vi "CANOpen Addon RT Driver VI.vi"(7 "Operation":T1, 11 "Device Reference in":T2 format="%.0x") -> (0 "Error Code":i32)   [LabVIEW 2013, in "CANOpen Addon Custom Device.lvlib"]
uses:
  CANOpen Addon Custom Device.lvlib
  <vilib>/NI Veristand/Custom Device API/Custom Device Item Ref.ctl
  <vilib>/NI Veristand/Custom Device API/Hardware Interface Driver VI Operation.ctl
  SubVIS/Inline Async API/_Controls/Async VI Control_Parameters Cluster.ctl
  SubVIS/Error Handling API/_Controls/VS Errors_Error Handling Cluster.ctl
  SubVIS/CANOpen_Settings.ctl
  SubVIS/CANOpen_Node Settings.ctl
  Shared Code/CANOpen_Bus Settings.ctl
  Shared Code/CANOpen Interface Name.ctl
  <vilib>/CANopenLib/CANOPEN.llb/CANopen BaudRate.ctl
  SubVIS/CANOpen_Node Message Settings.ctl
  Shared Code/CANOpen_PDO Settings.ctl
  Shared Code/CANOpen_PDO Parameter Settings.ctl
  Shared Code/CANOpen_PDO Data Type.ctl
  System Explorer/SubVIs/CANopen Byte Order.ctl
  Shared Code/CANOpen_SDO Settings.ctl
  SubVIS/CANOpen_NMT Settings.ctl
  Async VIs/CANOpen_Main/SubVIs/CanOpen_NMT_Config.ctl
  Async VIs/CANOpen_Main/SubVIs/CanOpen_NMT_Static detect.ctl
  Async VIs/CANOpen_Main/SubVIs/CanOpen_Main Node Ids.ctl
  SubVIS/CANOpen_VS Data Refs.ctl
  <vilib>/NI Veristand/Custom Device API/Data Reference.ctl
  <vilib>/NI Veristand/Custom Device API/Block Data Reference.ctl
  SubVIS/CANOpen_VS Bidirectional Data Refs.ctl
  SubVIS/CANOpen_VS SDOs Data Refs.ctl
  Async VIs/CANOpen_Main/SubVIs/CanOpen_SDO Dynamic queue.ctl
  Shared Code/CANOpen_SDO queue W data.ctl
  Shared Code/CANOpen_SDO queue mode.ctl
  Shared Code/CANOpen_PDO Data Type in queue.ctl
  SubVIS/CANOpen_VS Status Management Data Refs.ctl
  Async VIs/CANOpen_Main/SubVIs/CanOpen_NMT_HWOut_ChannelPairs.ctl
  Async VIs/CANOpen_Main/SubVIs/CanOpen_NMT_HWIn_ChannelPairs.ctl
  SubVIS/CANOpen_Get xPDO Data Refs.vi
  Shared Code/CANOpen_Get Node ID from Name.vi
  SubVIS/CANOpen_Get SDOs Settings.vi
  SubVIS/CANOpen_Get Dynamic SDOs Settings.vi
  SubVIS/CANOpen_NMR Read config.vi
  SubVIS/CANOpen_SetGet Bus Settings.vi
  SubVIS/CANOpen_Get Section References by GUID.vi
  SubVIS/CANOpen_Initialize VS Data Refs.vi
  SubVIS/CANOpen_Get Section References by GUID for SDOs.vi
  SubVIS/CANOpen_Get Section References by GUID for NMT.vi
  <vilib>/NI Veristand/Custom Device API/NI VeriStand - Set Channel Value by Data Reference.vi
  <vilib>/NI Veristand/Custom Device API/NI VeriStand - Get Channel Value by Data Reference.vi
  SubVIS/CANOpen_SDO List RW.vi
  SubVIS/CANOpen_SDO Read RW.vi
  SubVIS/CANOpen_SDO Write RW.vi
  <vilib>/NI Veristand/Custom Device API/NI VeriStand - Get Channel Values by Block Data Reference.vi
  <vilib>/NI Veristand/Custom Device API/NI VeriStand - Set Channel Values by Block Data Reference.vi
  SubVIS/Error Handling API/Print/VS Errors_Display and Log Custom Device Error.vi
  Shared Code/CANOpen_Get PDO Channel from Name.vi
  Shared Code/CANOpen_SetGet PDO Parameter Settings.vi
  SubVIS/CANOpen_SetGet NMT Settings.vi
  SubVIS/CANOpen_Initialize VS BiDirectional Data Refs.vi
  SubVIS/CANOpen_Search Channel Ref.vi
  SubVIS/CANOpen_Search Channel Refs.vi
  SubVIS/CANOpen_Initialize VS NMT Data Refs.vi
  SubVIS/CANOpen_SDO Update status channels Dyn Read.vi
  SubVIS/CANOpen_SDO Update status channels Dyn Write.vi
  <vilib>/NI Veristand/Custom Device Tools/Custom Device Utility Library/NI VeriStand - Search for Item.vi
  <vilib>/NI Veristand/Custom Device Tools/Custom Device Utility Library/NI VeriStand - Search for All Items by GUID.vi
  <vilib>/NI Veristand/Custom Device API/NI VeriStand - Get Item Property.vi
  <vilib>/NI Veristand/Custom Device API/Get Item Property (Variant).vi
  Shared Code/CANOpen Addon GUID Lookup Global.vi
  <vilib>/NI Veristand/Custom Device API/NI VeriStand - Get Item Children.vi
  <vilib>/NI Veristand/Custom Device Tools/Custom Device Utility Library/NI VeriStand - Search for Item by GUID.vi
  <vilib>/NI Veristand/Custom Device API/NI VeriStand - Get Channel Data Reference.vi
  <vilib>/NI Veristand/Custom Device API/NI VeriStand - Get Channel Block Data References.vi
  <vilib>/NI Veristand/Custom Device API/Global Data Refs.vi
  <vilib>/Utility/error.llb/Simple Error Handler.vi
  <vilib>/NI Veristand/Custom Device API/Custom Device API.lvlib
  <vilib>/NI Veristand/Custom Device API/Custom Device Item Info.ctl
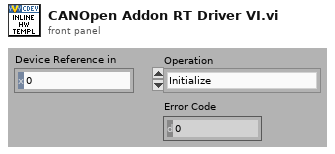
[diagram p1: front panel]
types:
  T1 = typedef "Custom Device API.lvlib/Hardware Interface Driver VI Operation.ctl" = enum16{"Initialize", "Start", "Read Data from HW", "Write Data to HW", "Close"}
  T2 = typedef "Custom Device API.lvlib/Custom Device Item Ref.ctl" = u64
  T3 = typedef "CANOpen Addon Custom Device.lvlib/VS Errors_Error Handling Cluster.ctl" = cluster{"Error Process Q":refnum<queue>, "Process Qs":refnum<queue>[]}
  T4 = typedef "CANOpen_Settings.ctl" = cluster{"Driver Settings":T5, "Data References":T19, "Bus Commands":T22, "SDO Asynch":T23, "Status NMT":T24}
  T5 = typedef "CANOpen_Node Settings.ctl" = cluster{"CANOpen Bus Settings":T6, "Nodes":T9[], "Node Ids":T18}
  T6 = typedef "CANOpen Addon Custom Device.lvlib/CANOpen_Bus Settings.ctl" = cluster{"CANOpen Interface Name":T7, "Baud Rate":T8, "Termination":bool, "Sync Period (ms)":i64, "Enable 9881":bool, "RIO Device":u16, "Enable SYNC":bool, "Scan & Print":bool}
  T7 = typedef "CANOpen Addon Custom Device.lvlib/CANOpen Interface Name.ctl" = u32
  T8 = typedef "CANopen BaudRate.ctl" = u32
  T9 = typedef "CANOpen_Node Message Settings.ctl" = cluster{"RPDOs":T10[], "TPDOs":T10[], "Node ID":u8, "SDOs":T14[], "Dynamic SDOs":T14[], "NMT":T15}
  T10 = typedef "CANOpen Addon Custom Device.lvlib/CANOpen_PDO Settings.ctl" = cluster{"Parameters":T11[], "PDO Channel":u8, "Start Index":u32, "Length":u32}
  T11 = typedef "CANOpen Addon Custom Device.lvlib/CANOpen_PDO Parameter Settings.ctl" = cluster{"Parameter Name":string, "Scale Factor":dbl, "Scale Offset":dbl, "Byte Offset":u8, "Bit Offset":u8, "Data Type":T12, "Byte Order":T13}
  T12 = typedef "CANOpen Addon Custom Device.lvlib/CANOpen_PDO Data Type.ctl" = enum16{"U8", "U16", "U32", "I8", "I16", "I32", "Single", "Double", "Boolean"}
  T13 = typedef "CANOpen Addon Custom Device.lvlib/CANopen Byte Order.ctl" = enum16{"big-endian network order", "little-endian"}
  T14 = typedef "CANOpen Addon Custom Device.lvlib/CANOpen_SDO Settings.ctl" = cluster{"Object Index":u16, "Sub-Index (0)":u8, "Block Data":u8[], "Name":string}
  T15 = typedef "CANOpen Addon Custom Device.lvlib/CANOpen_NMT Settings.ctl" = cluster{"Node run state":u16, "Emergency":bool, "HB NG":T16, "Delay for opp. state (ms)":dbl, "Node init static SDO state":u16, "Stop and Reset on Shutdown":bool}
  T16 = typedef "CANOpen Addon Custom Device.lvlib/CanOpen_NMT_Config.ctl" = cluster{"Mode":T17, "Update Time":u16, "Static detect in None":T17}
  T17 = typedef "CANOpen Addon Custom Device.lvlib/CanOpen_NMT_Static detect.ctl" = enum16{"None", "HB", "NG"}
  T18 = typedef "CANOpen Addon Custom Device.lvlib/CanOpen_Main Node Ids.ctl" = u8[]
  T19 = typedef "CANOpen_VS Data Refs.ctl" = cluster{"Hardware Input":cluster{"FIFO":refnum<k33>, "Channel Pairs":cluster{"Chan Refs":T20[], "Prev. Values":dbl[]}}, "Hardware Output":cluster{"FIFO":refnum<k33>, "Channel Pairs":cluster{"Block Refs":T21[], "Prev. Values":dbl[]}}}
  T20 = typedef "Custom Device API.lvlib/Data Reference.ctl" = i32
  T21 = typedef "Custom Device API.lvlib/Block Data Reference.ctl" = cluster{"Data Reference":T20, "Offset":i32, "Length":i32}
  T22 = typedef "CANOpen_VS Bidirectional Data Refs.ctl" = cluster{"Hardware Output":cluster{"FIFO":refnum<k33>, "Channel Pairs":cluster{"Chan Refs":T20[], "Prev. Values":dbl[]}}, "Hardware Input":cluster{"FIFO":refnum<k33>}}
  T23 = typedef "CANOpen Addon Custom Device.lvlib/CANOpen_VS SDOs Data Refs.ctl" = cluster{"List SDO":cluster{"FIFO Req":refnum<k33>, "Req Chan.":cluster{"Chan Refs":T20[], "NodeIndex":dbl[]}, "FIFO Resp":refnum<k33>, "Resp Chan.":cluster{"Chan Refs":T20[]}, "Node IDs":u8[], "FIFO array":dbl[]}, "HW Dyn Write":cluster{"FIFO Req":refnum<k33>, "FIFO Resp":refnum<k33>, "Req Chan.":cluster{"Chan Refs":T20[], "Node IDs":u8[]}, "Resp Chan.":cluster{"Chan Refs":T20[]}}, "HW Dyn Read":cluster{"FIFO Req":refnum<k33>, "FIFO Resp":refnum<k33>, "Req Chan.":cluster{"Chan Refs":T20[], "Node IDs":u8[]}, "Resp Chan.":cluster{"Chan Refs":T20[]}}}
  T24 = typedef "CANOpen Addon Custom Device.lvlib/CANOpen_VS Status Management Data Refs.ctl" = cluster{"Hardware Output":cluster{"FIFO":refnum<k33>, "Channel Pairs":T25}, "Hardware Input":cluster{"FIFO":refnum<k33>, "Channel Pairs":T26}}
  T25 = typedef "CANOpen Addon Custom Device.lvlib/CanOpen_NMT_HWOut_ChannelPairs.ctl" = cluster{"Chan Refs":T21[], "Prev. Values":dbl[], "Node index":dbl[]}
  T26 = typedef "CANOpen Addon Custom Device.lvlib/CanOpen_NMT_HWIn_ChannelPairs.ctl" = cluster{"Chan Refs":T20[], "Prev. Values":dbl[], "Node index":dbl[]}
  T27 = cluster{"Device Error":errorcluster, "Error Handling Cluster":T3, "VI Ref In":refnum<vi>[], "CD Settings":T4, "FPGA Session":u32}
  T28 = typedef "CANOpen Addon Custom Device.lvlib/Async VI Control_Parameters Cluster.ctl" = cluster{"Parameter Name":string, "Initial Settings":variant}
  T29 = typedef "Custom Device API.lvlib/Custom Device Item Info.ctl" = cluster{"Name":string, "Is Channel":bool, "GUID":string, "Is Waveform":bool}
  T30 = cluster{"Chan Refs":T20[], "Previous Chan Values":dbl[]}
  T31 = cluster{"Block Refs":T21[], "Prev. Values":dbl[]}
  T32 = cluster{"Block Data Refs":T21[], "Previous Chan Values":dbl[]}
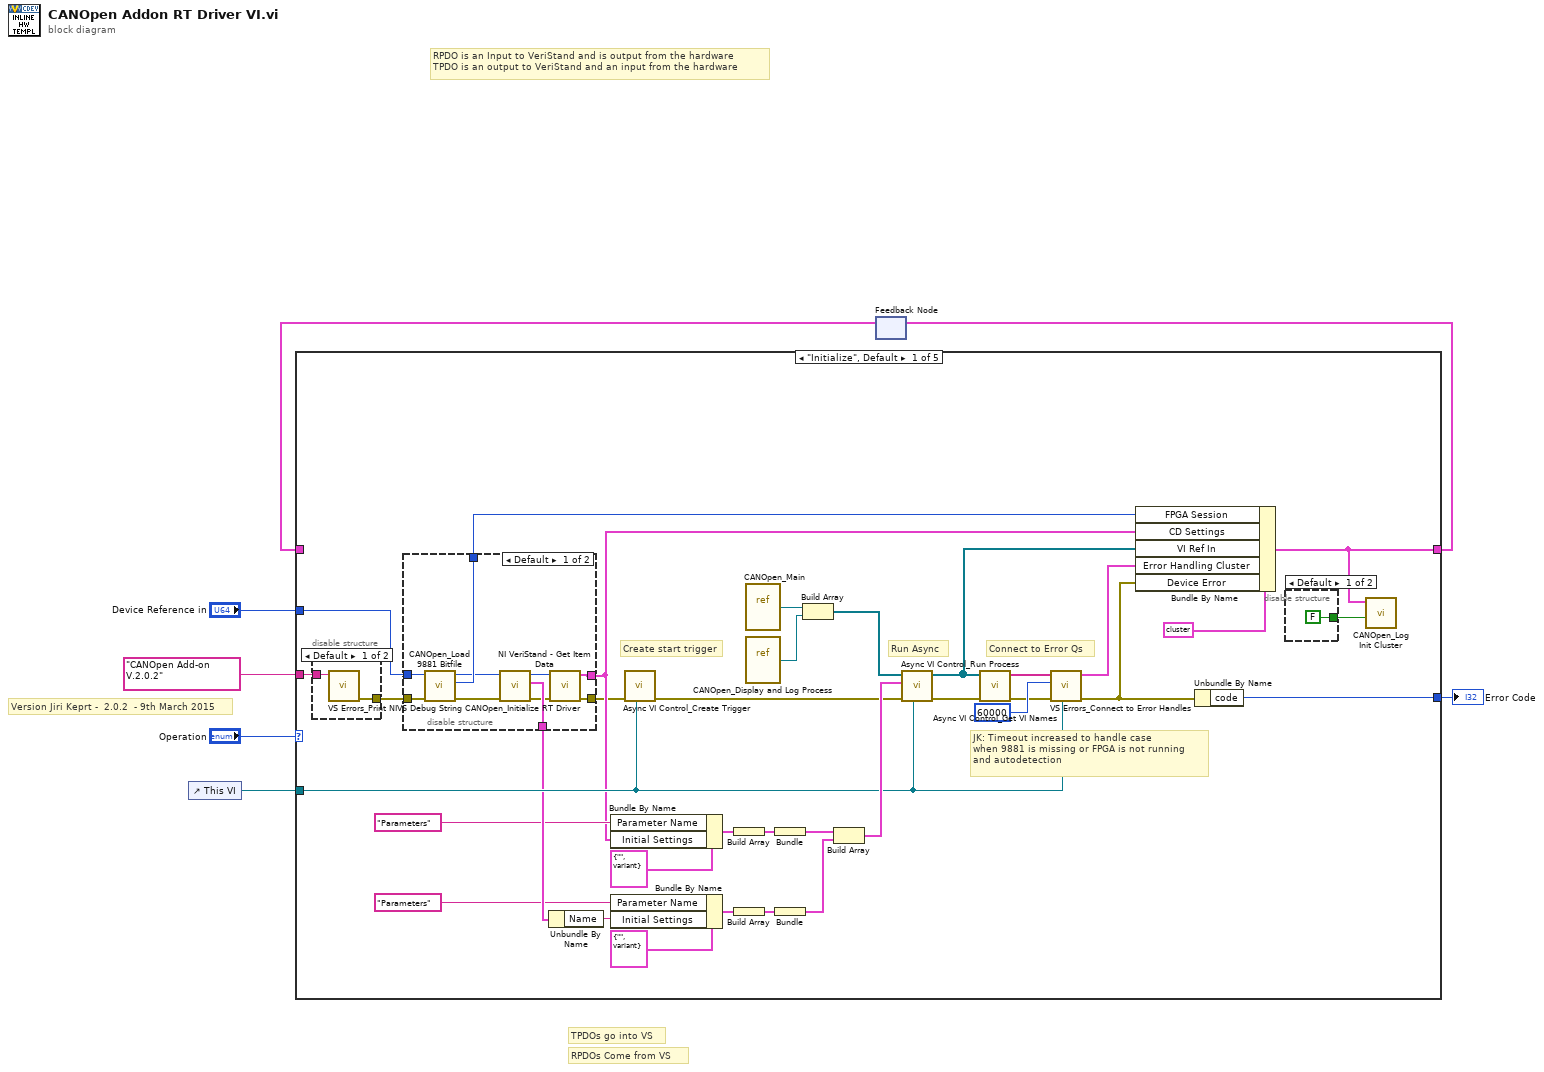
[diagram p0: block diagram]
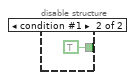
[diagram p2: hidden frame]
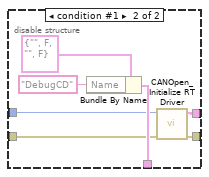
[diagram p4: hidden frame]
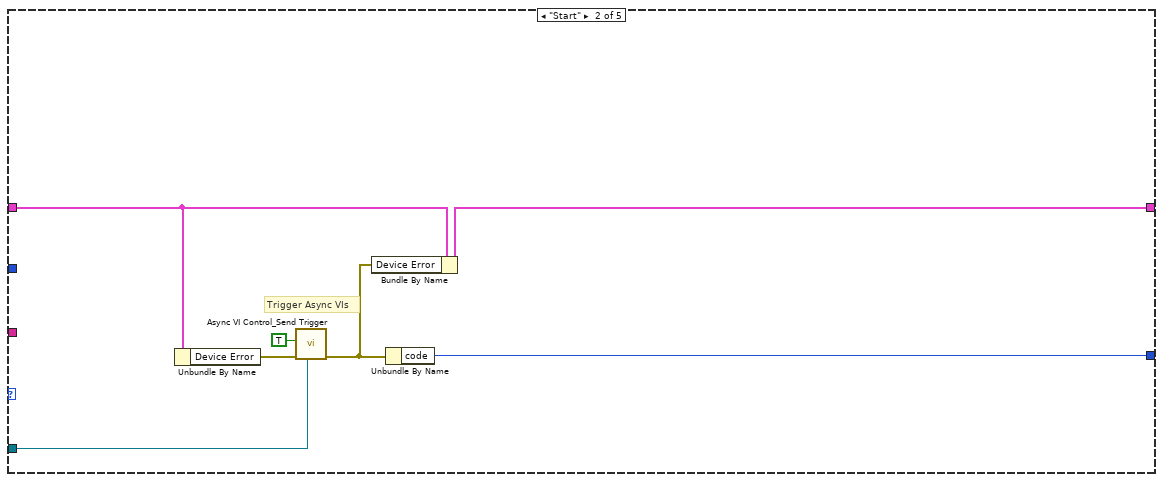
[diagram p5: hidden frame]
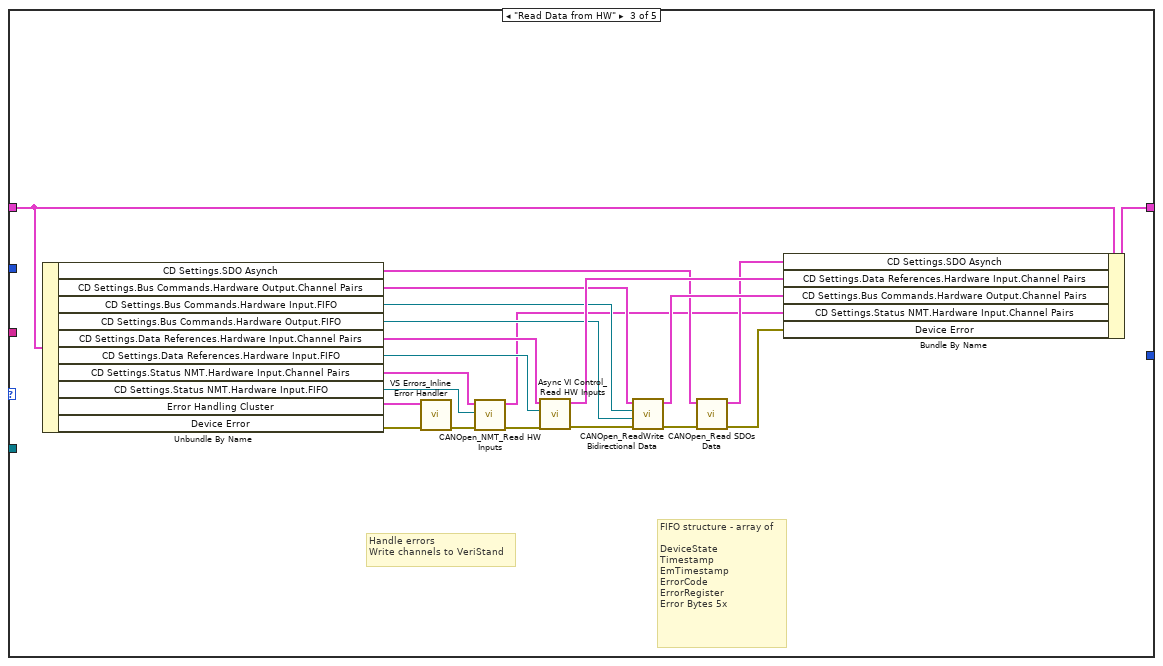
[diagram p6: hidden frame]
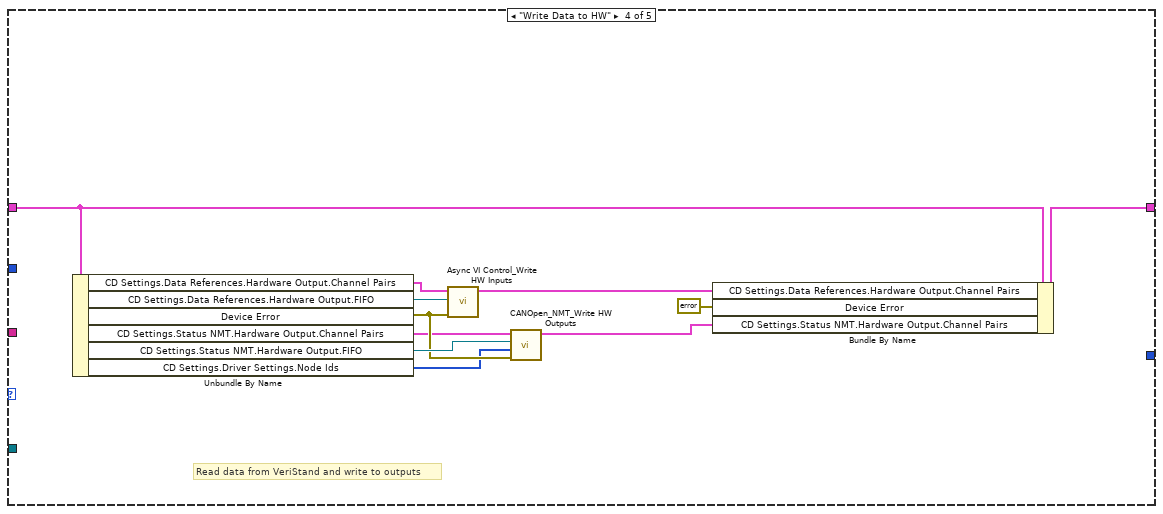
[diagram p7: hidden frame]
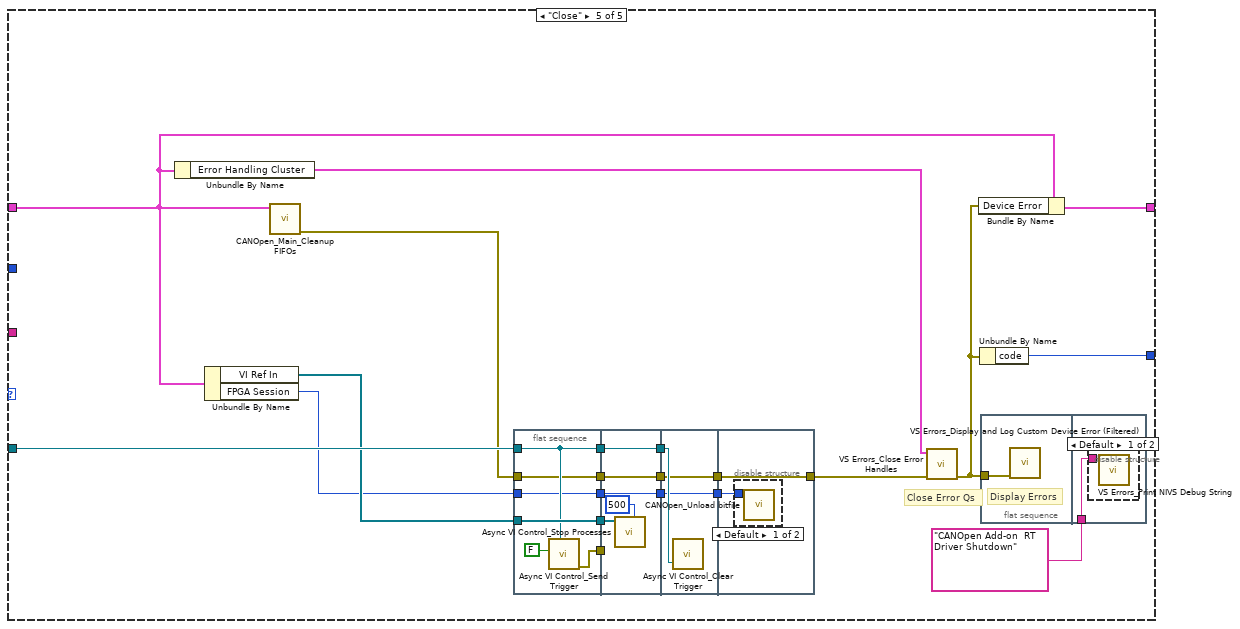
[diagram p8: hidden frame]
diagram:
  # "Version Jiri Keprt -  2.0.2  - 9th March 2015"
  # "RPDO is an Input to VeriStand and is output from the hardware\nTPDO is an output to VeriStand and an input from the hardware"
  # "RPDOs Come from VS"
  # "TPDOs go into VS"
  n1 = control-ref of="This VI"() -> (w1:refnum<vi>)
  n2 = feedback #1() -> (w5:T27)  [unwired: 1 out]
  n3 = case shown="\"Initialize\", Default" "Operation" {
    tunnel: [w19 w66 w87 w98 w122] -> w6
    tunnel: w5 -> [_ w67 w88 w99 w109]
    tunnel: "Device Reference in" -> [w15 _ _ _ _]
    tunnel: [w42 w65 _ _ w121] -> w3
    tunnel: "CANOpen Add-on  V.2.0.2" ("Debug String") -> [w41 _ _ _ _]
    tunnel: w1 -> [w30 w64 _ _ w113]
    frame "Initialize", Default {
      # "JK: Timeout increased to handle case\nwhen 9881 is missing or FPGA is not running\nand autodetection"
      # "Connect to Error Qs"
      # "Run Async"
      # "Create start trigger"
      n4 = disable-structure shown="Default" {
        disable-tunnel: w41 -> [w46 _]
        disable-tunnel: [w45 _] -> w13
        frame condition #0 (active) {
          n5 = call "VS Errors_Print NIVS Debug String.vi"("Debug String"=w46) -> ("error out"=w45:errorcluster)  [unwired: 9 in]
        }
        frame condition #1 {
        }
      }
      n6 = disable-structure shown="Default" {
        disable-tunnel: [w56 w61] -> w29
        disable-tunnel: [w54 w57] -> w17
        disable-tunnel: w15 -> [w53 w58]
        disable-tunnel: [w52 _] -> w14
        disable-tunnel: w13 -> [w50 w59]
        disable-tunnel: [w47 w60] -> w8
        frame condition #0 (active) {
          n7 = call "CANOpen_Load 9881 Bitfile.vi"("error in (no error)"=w50, "Item Ref in"=w53) -> ("error out"=w49:errorcluster, "FPGA Session"=w52:u32, "Item Ref out"=w51:T2)  [unwired: 7 in]
          n8 = call <vilib>:"NI VeriStand - Get Item Data.vi"("error in (no error)"=w49, "Item Ref in"=w51) -> ("error out"=w48:errorcluster, "Item Info"=w56:T29, "Item Ref out"=w55:T2)  [unwired: 6 in, 1 out]
          n9 = call "CANOpen_Initialize RT Driver.vi"("error in (no error)"=w48, "Device Reference in"=w55) -> ("error out"=w47:errorcluster, "Configuration Cluster"=w54:T4)  [unwired: 8 in]
        }
        frame condition #1 {
          n10 = Bundle By Name(cluster=T29 {"Name"="", "Is Channel"=FALSE, "GUID"="", "Is Waveform"=FALSE} ("Item Info"), "Name"="DebugCD") -> (w61:T29)
          n11 = call "CANOpen_Initialize RT Driver.vi"("error in (no error)"=w59, "Device Reference in"=w58) -> ("error out"=w60:errorcluster, "Configuration Cluster"=w57:T4)  [unwired: 8 in]
        }
      }
      n12 = Unbundle By Name(w29) -> ("Name"=w28:string)
      n13 = Bundle By Name(cluster=T28 {"Parameter Name"="", "Initial Settings"=variant} ("Parameters"), "Parameter Name"="Parameters", "Initial Settings"=w17) -> (w23:T28)
      n14 = Bundle By Name(cluster=T28 {"Parameter Name"="", "Initial Settings"=variant} ("Parameters"), "Parameter Name"="Parameters", "Initial Settings"=w28) -> (w37:T28)
      n15 = call "Async VI Control_Create Trigger.vi"("This VI"=w30, "error in (no error)"=w8) -> ("error out"=w12:errorcluster)  [unwired: 9 in]
      n16 = Build Array(w23) -> (w24:T28[])
      n17 = Build Array(w37) -> (w38:T28[])
      n18 = vi-ref "CANOpen_Main.vi"() -> (w35:refnum<vi>)
      n19 = vi-ref "CANOpen_Display and Log Process.vi"() -> (w31:refnum<vi>)
      n20 = Bundle ("Display and Log Process Parameters")(w24) -> (w20:cluster{T28[]})  [unwired: 1 in]
      n21 = Bundle ("Display and Log Process Parameters")(w38) -> (w39:cluster{T28[]})  [unwired: 1 in]
      n22 = Build Array(w35, w31) -> (w32:refnum<vi>[])
      n23 = Build Array(w20, w39) -> (w40:cluster{T28[]}[])
      n24 = call "Async VI Control_Run Process.vi"("Parent VI"=w30, "error in (no error)"=w12, "Initial Parameters"=w40, "VI Ref In"=w32) -> ("error out"=w11:errorcluster, "VI Ref In"=w25:refnum<vi>[])  [unwired: 6 in]
      n25 = call "Async VI Control_Get VI Names.vi"("error in"=w11, "VI References"=w25) -> ("error out"=w10:errorcluster, "Clone Names"=w33:string[])  [unwired: 8 in]
      n26 = call "VS Errors_Connect to Error Handles.vi"("Parent"=w30, "error in"=w10, "Timeout (ms)"=u16 60000, "Process Names"=w33) -> ("error out"=w9:errorcluster, "Error Handling Cluster"=w26:T3)  [unwired: 6 in]
      n27 = Bundle By Name(cluster=T27 {"Device Error"={"status"=FALSE, "code"=0, "source"=""}, "Error Handling Cluster"={"Error Process Q"=refnum, "Process Qs"=[]}, "VI Ref In"=[], "CD Settings"={"Driver Settings"={"CANOpen Bus Settings"={"CANOpen Interface Name"=0, "Baud Rate"=0, "Termination"=FALSE, "Sync Period (ms)"=0, "Enable 9881"=FALSE, "RIO Device"=0, "Enable SYNC"=FALSE, "Scan & Print"=FALSE}, "Nodes"=[], "Node Ids"=[]}, "Data References"={"Hardware Input"={"FIFO"=refnum, "Channel Pairs"={"Chan Refs"=[], "Prev. Values"=[]}}, "Hardware Output"={"FIFO"=refnum, "Channel Pairs"={"Block Refs"=[], "Prev. Values"=[]}}}, "Bus Commands"={"Hardware Output"={"FIFO"=refnum, "Channel Pairs"={"Chan Refs"=[], "Prev. Values"=[]}}, "Hardware Input"={"FIFO"=refnum}}, "SDO Asynch"={"List SDO"={"FIFO Req"=refnum, "Req Chan."={"Chan Refs"=[], "NodeIndex"=[]}, "FIFO Resp"=refnum, "Resp Chan."={"Chan Refs"=[]}, "Node IDs"=[], "FIFO array"=[]}, "HW Dyn Write"={"FIFO Req"=refnum, "FIFO Resp"=refnum, "Req Chan."={"Chan Refs"=[], "Node IDs"=[]}, "Resp Chan."={"Chan Refs"=[]}}, "HW Dyn Read"={"FIFO Req"=refnum, "FIFO Resp"=refnum, "Req Chan."={"Chan Refs"=[], "Node IDs"=[]}, "Resp Chan."={"Chan Refs"=[]}}}, "Status NMT"={"Hardware Output"={"FIFO"=refnum, "Channel Pairs"={"Chan Refs"=[], "Prev. Values"=[], "Node index"=[]}}, "Hardware Input"={"FIFO"=refnum, "Channel Pairs"={"Chan Refs"=[], "Prev. Values"=[], "Node index"=[]}}}}, "FPGA Session"=0}, "FPGA Session"=w14, "CD Settings"=w17, "VI Ref In"=w25, "Error Handling Cluster"=w26, "Device Error"=w9) -> (w19:T27)
      n28 = Unbundle By Name(w9) -> ("code"=w42:i32)
      n29 = disable-structure shown="Default" {
        disable-tunnel: [FALSE ("Write?") TRUE ("Write?")] -> w18
        frame condition #0 (active) {
        }
        frame condition #1 {
        }
      }
      n30 = call "CANOpen_Log Init Cluster.vi"("Write?"=w18, "cluster 2"=w19) -> ()  [unwired: 8 in, 2 out]
    }
    frame "Start" {
      # "Trigger Async VIs"
      n31 = Unbundle By Name(w67) -> ("Device Error"=w68:errorcluster)
      n32 = call "Async VI Control_Send Trigger.vi"("Parent VI"=w64, "error in (no error)"=w68, "notification"=TRUE) -> ("error out"=w69:errorcluster)  [unwired: 8 in]
      n33 = Bundle By Name(cluster=w67, "Device Error"=w69) -> (w66:T27)
      n34 = Unbundle By Name(w69) -> ("code"=w65:i32)
    }
    frame "Read Data from HW" {
      # "FIFO structure - array of\n\nDeviceState\nTimestamp\nEmTimestamp\nErrorCode\nErrorRegister\nError Bytes 5x"
      # "Handle errors\nWrite channels to VeriStand"
      n35 = Unbundle By Name(w88) -> ("CD Settings.SDO Asynch"=w80:T23, "CD Settings.Bus Commands.Hardware Output.Channel Pairs"=w84:cluster{"Chan Refs":T20[], "Prev. Values":dbl[]}, "CD Settings.Bus Commands.Hardware Input.FIFO"=w83:refnum<k33>, "CD Settings.Bus Commands.Hardware Output.FIFO"=w82:refnum<k33>, "CD Settings.Data References.Hardware Input.Channel Pairs"=w89:cluster{"Chan Refs":T20[], "Prev. Values":dbl[]}, "CD Settings.Data References.Hardware Input.FIFO"=w91:refnum<k33>, "CD Settings.Status NMT.Hardware Input.Channel Pairs"=w73:T26, "CD Settings.Status NMT.Hardware Input.FIFO"=w74:refnum<k33>, "Error Handling Cluster"=w77:T3, "Device Error"=w78:errorcluster)
      n36 = call "VS Errors_Inline Error Handler.vi"("error in"=w78, "Error Handling Cluster"=w77) -> ("error out"=w75:errorcluster)  [unwired: 9 in]
      n37 = call "CANOpen_NMT_Read HW Inputs.vi"("error in"=w75, "Hardware Input FIFO"=w74, "Channel Pairs"=w73) -> ("error out"=w76:errorcluster, "Channel Pairs Out"=w71:T26)  [unwired: 6 in, 1 out]
      n38 = call "Async VI Control_Read HW Inputs.vi"("error in"=w76, "Hardware Input FIFO"=w91, "Channel Pairs"=w89) -> ("error out"=w86:errorcluster, "Channel Pairs Out"=w90:T30)  [unwired: 6 in, 1 out]
      n39 = call "CANOpen_ReadWrite Bidirectional Data.vi"("error in"=w86, "Hardware Output FIFO"=w82, "Hardware Input FIFO"=w83, "Channel Pairs"=w84) -> ("error out"=w81:errorcluster, "Channel Pairs Out"=w85:T30)  [unwired: 5 in, 1 out]
      n40 = call "CANOpen_Read SDOs Data.vi"("error in"=w81, "SDO Asynch"=w80) -> ("error out"=w72:errorcluster, "SDO Asynch out"=w79:T23)  [unwired: 8 in]
      n41 = Bundle By Name(cluster=w88, "CD Settings.SDO Asynch"=w79, "CD Settings.Data References.Hardware Input.Channel Pairs"=w90, "CD Settings.Bus Commands.Hardware Output.Channel Pairs"=w85, "CD Settings.Status NMT.Hardware Input.Channel Pairs"=w71, "Device Error"=w72) -> (w87:T27)
    }
    frame "Write Data to HW" {
      # "Read data from VeriStand and write to outputs"
      n42 = Unbundle By Name(w99) -> ("CD Settings.Data References.Hardware Output.Channel Pairs"=w101:T31, "CD Settings.Data References.Hardware Output.FIFO"=w102:refnum<k33>, "Device Error"=w96:errorcluster, "CD Settings.Status NMT.Hardware Output.Channel Pairs"=w95:T25, "CD Settings.Status NMT.Hardware Output.FIFO"=w97:refnum<k33>, "CD Settings.Driver Settings.Node Ids"=w94:T18)
      n43 = call "Async VI Control_Write HW Inputs.vi"("error in"=w96, "Hardware Output FIFO"=w102, "Channel Pairs"=w101) -> ("Channel Pairs"=w92:T32)  [unwired: 6 in, 2 out]
      n44 = call "CANOpen_NMT_Write HW Outputs.vi"("error in"=w96, "Node Ids"=w94, "Hardware Output FIFO"=w97, "Channel Pairs"=w95) -> ("Channel Pairs"=w93:T25)  [unwired: 5 in, 2 out]
      n45 = Bundle By Name(cluster=w99, "CD Settings.Data References.Hardware Output.Channel Pairs"=w92, "Device Error"=errorcluster {"status"=FALSE, "code"=0, "source"=""}, "CD Settings.Status NMT.Hardware Output.Channel Pairs"=w93) -> (w98:T27)
    }
    frame "Close" {
      # "Close Error Qs"
      n46 = Unbundle By Name(w109) -> ("Error Handling Cluster"=w111:T3)
      n47 = Unbundle By Name(w109) -> ("VI Ref In"=w110:refnum<vi>[], "FPGA Session"=w106:u32)
      n48 = call "CANOpen_Main_Cleanup FIFOs.vi"("Data"=w109) -> ("error out"=w108:errorcluster)  [unwired: 10 in]
      n49 = flat-sequence {
        tunnel: [w129] -> w119
        tunnel: [w128] -> w118
        tunnel: [w127] -> w117
        tunnel: [w126] -> w116
        tunnel: w108 -> [w126]
        tunnel: w113 -> [w128]
        tunnel: w110 -> [w129]
        tunnel: w106 -> [w124]
        tunnel: [w124] -> w105
        tunnel: w119 -> [w134]
        tunnel: [w133] -> w115
        tunnel: w118 -> [w133]
        tunnel: w117 -> [_]
        tunnel: [w132] -> w114
        tunnel: w116 -> [w132]
        tunnel: w105 -> [w130]
        tunnel: [w130] -> w104
        tunnel: w115 -> [w137]
        tunnel: w114 -> [w136]
        tunnel: [w136] -> w107
        tunnel: w104 -> [w135]
        tunnel: [w135] -> w103
        tunnel: [w139] -> w112
        tunnel: w107 -> [w139]
        tunnel: w103 -> [w138]
        frame #0 {
          n50 = call "Async VI Control_Send Trigger.vi"("Parent VI"=w128, "notification"=FALSE) -> ("error out"=w127:errorcluster)  [unwired: 9 in]
        }
        frame #1 {
          n51 = call "Async VI Control_Stop Processes.vi"("Iterations"=500, "VI Refs"=w134) -> ()  [unwired: 10 in]
        }
        frame #2 {
          n52 = call "Async VI Control_Clear Trigger.vi"("Parent VI"=w137) -> ()  [unwired: 10 in, 1 out]
        }
        frame #3 {
          n53 = disable-structure shown="Default" {
            disable-tunnel: w138 -> [w140 _]
            frame condition #0 (active) {
              n54 = call "CANOpen_Unload bitfile.vi"("Session"=w140) -> ()  [unwired: 11 in]
            }
            frame condition #1 {
            }
          }
        }
      }
      n55 = call "VS Errors_Close Error Handles.vi"("error in"=w112, "Error Handling Cluster"=w111) -> ("error out"=w123:errorcluster)  [unwired: 9 in]
      n56 = Bundle By Name(cluster=w109, "Device Error"=w123) -> (w122:T27)
      n57 = Unbundle By Name(w123) -> ("code"=w121:i32)
      n58 = flat-sequence {
        tunnel: w123 -> [w141]
        tunnel: "CANOpen Add-on  RT Driver Shutdown" ("Debug String") -> [w142]
        frame #0 {
          # "Display Errors"
          n59 = call "VS Errors_Display and Log Custom Device Error (Filtered).vi"("error in (no error)"=w141) -> ()  [unwired: 11 in]
        }
        frame #1 {
          n60 = disable-structure shown="Default" {
            disable-tunnel: w142 -> [w143 _]
            frame condition #0 (active) {
              n61 = call "VS Errors_Print NIVS Debug String.vi"("Debug String"=w143) -> ()  [unwired: 9 in, 1 out]
            }
            frame condition #1 {
            }
          }
        }
      }
    }
  }
  "Error Code" <- w3
  n62 = feedback-in #1(w6) -> ()
